vi "VerticalSpeedIndicator.vi"(6 "SignalSource":T2(ring), 7 "ScaleUnit(F=m/s; T=Ft/min/100)":bool, 8 "error in (no error)":errorcluster caption="Fehler (Eingang, kein Fehler)", 11 "SBG Data Cluster":T1) -> (0 "error out":errorcluster caption="Fehler (Ausgang)", 2 "VerticalSpeedDigital":dbl format="%.1f", 3 "VerticalSpeedIndicator":picture)   [LabVIEW 2023]
uses:
  SBG Data Cluster.ctl
  <vilib>/picture/picture.llb/imagedata.ctl
  <vilib>/Utility/miscctls.llb/LVBoundsTypeDef.ctl
panel:
  in  "Transparent":picture caption="Neue Grafik"
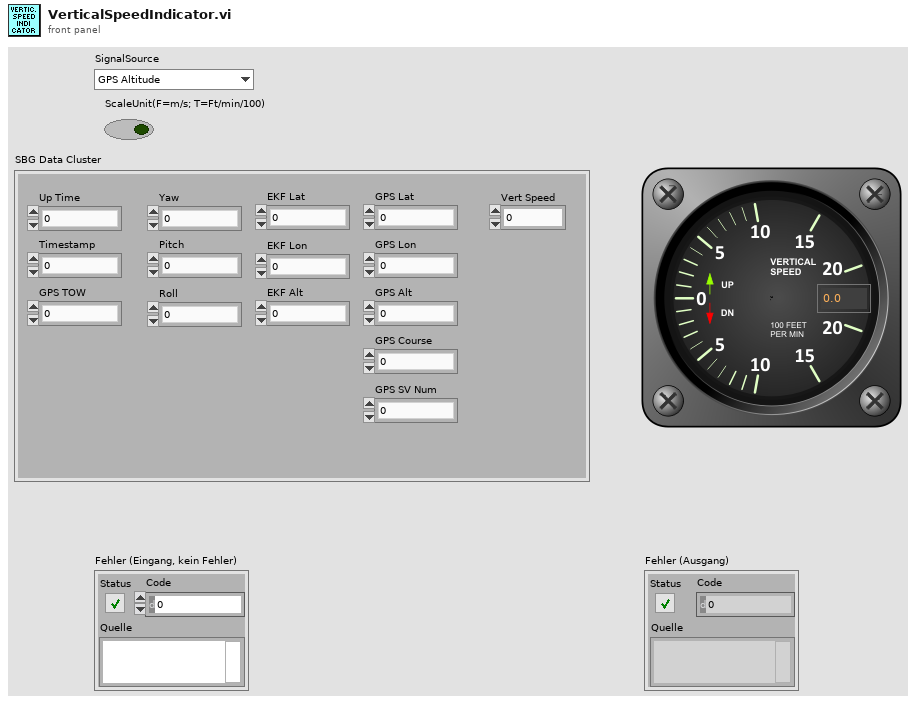
[diagram p1: front panel]
types:
  T1 = typedef "SBG Data Cluster.ctl" = cluster{"Up Time":u32, "Timestamp":u32, "Yaw":sgl, "Pitch":sgl, "Roll":sgl, "EKF Lat":dbl, "EKF Lon":dbl, "EKF Alt":dbl, "GPS Lat":dbl, "GPS Lon":dbl, "GPS Alt":dbl, "GPS Course":sgl, "GPS SV Num":u8, "GPS TOW":u32, "Vert Speed":dbl}
  T2 = enum16{"GPS Altitude", "Baro absolute Altitude", "Baro Vario"}
  T3 = typedef "LVBoundsTypeDef.ctl" = cluster{"Width":u32, "Height":u32}
  T4 = typedef "imagedata.ctl" = cluster{"image type":i32, "image depth":i32, "image":u8[], "mask":u8[], "colors":u32[], "Rectangle":cluster{"left":i16, "top":i16, "right":i16, "bottom":i16}}
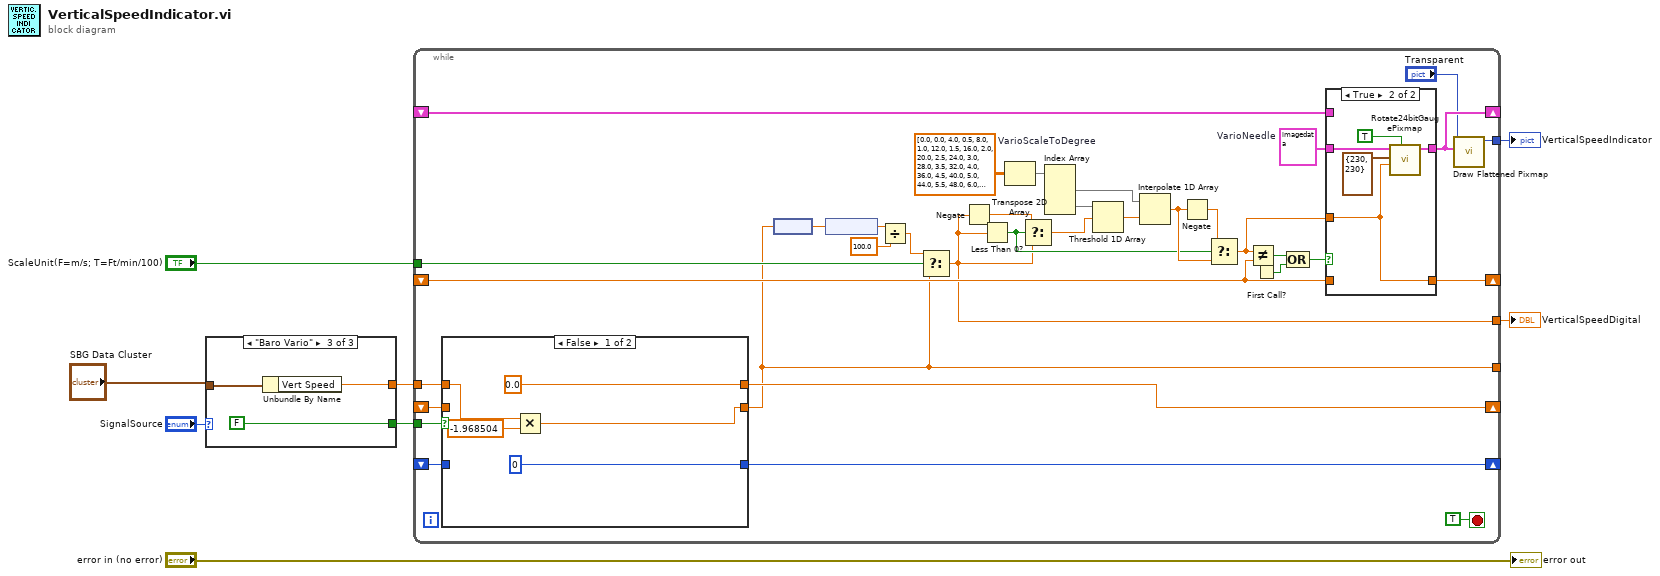
[diagram p0: block diagram]
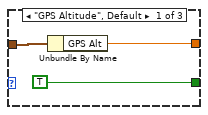
[diagram p2: hidden frame]
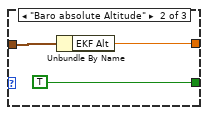
[diagram p3: hidden frame]
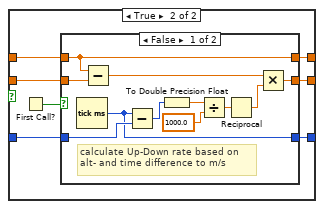
[diagram p4: hidden frame]
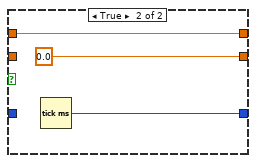
[diagram p5: hidden frame]
diagram:
  n1 = case shown="\"Baro Vario\"" "SignalSource" {
    tunnel: [TRUE TRUE FALSE] -> w3
    tunnel: "SBG Data Cluster" -> [w11 w14 w16]
    tunnel: [w10 w12 w15] -> w4
    frame "GPS Altitude", Default {
      n2 = Unbundle By Name(w11) -> ("GPS Alt"=w10:dbl)
    }
    frame "Baro absolute Altitude" {
      n3 = Unbundle By Name(w14) -> ("EKF Alt"=w12:dbl)
    }
    frame "Baro Vario" {
      n4 = Unbundle By Name(w16) -> ("Vert Speed"=w15:dbl)
    }
  }
  n5 = while {
    shift-right: [w50] -> _
    shift-left: _ -> [w44]
    shift-right: [w49] -> _
    shift-left: _ -> [w48]
    tunnel: [w46] -> w8
    tunnel: w4 -> [w23]
    tunnel: "ScaleUnit(F=m/s; T=Ft/min/100)" -> [w31]
    tunnel: [w18] -> w2
    tunnel: [w22] -> _
    shift-right: [w26] -> _
    shift-left: _ -> [w27]
    tunnel: w3 -> [w24]
    shift-right: [w21] -> _
    shift-left: _ -> [w20]
    stop <- TRUE stop-if-true
    w42 = dbl[][] [[0.0, 0.0], [4.0, 0.5], [8.0, 1.0], [12.0, 1.5], [16.0, 2.0], [20.0, 2.5], [24.0, 3.0], [28.0, 3.5], [32.0, 4.0], [36.0, 4.5], [40.0, 5.0], [44.0, 5.5], [48.0, 6.0], [52.0, 6.5], [56.0, 7.0], [60.0, 7.5], [64.0, 8.0], [68.0, 8.5], [72.0, 9.0], [76.0, 9.5], [80.0, 10.0], [88.0, 11.0], [96.0, 12.0], [104.0, 13.0], [112.0, 14.0], [120.0, 15.0], [128.0, 16.0], [136.0, 17.0], [144.0, 18.0], [152.0, 19.0], [160.0, 20.0]]  # VarioScaleToDegree
    w43 = T4 {"image type"=0, "image depth"=24, "image"=array[158700 elements], "mask"=[], "colors"=[], "Rectangle"={"left"=0, "top"=0, "right"=230, "bottom"=230}}  # VarioNeedle
    n6 = case shown="False" w24 {
      tunnel: w27 -> [_ w64]
      tunnel: [0.0 ("VerticalSpeed (m/s)") w63] -> w26
      tunnel: w23 -> [w55 w62]
      tunnel: [w53 w60] -> w22
      tunnel: [u32 0 ("millisecond timer value") w59] -> w21
      tunnel: w20 -> [_ w58]
      frame False {
        n7 = Multiply(x=w55, y=-1.968504) -> (x*y=w53:dbl)
      }
      frame True {
        n8 = First Call?() -> (First Call?: T/F=w61:bool)
        n9 = case shown="False" w61 {
          tunnel: w62 -> [w74 w78]
          tunnel: [w74 w78] -> w63
          tunnel: w64 -> [w75 _]
          tunnel: [w67 0.0] -> w60
          tunnel: [w72 w76] -> w59
          tunnel: w58 -> [w73 _]
          frame False {
            # "calculate Up-Down rate based on\nalt- and time difference to m/s"
            n10 = Tick Count (ms)() -> (millisecond timer value=w72:u32)
            n11 = Subtract(x=w74, y=w75) -> (x-y=w66:dbl)
            n12 = Subtract(x=w72, y=w73) -> (x-y=w71:u32)
            n13 = To Double Precision Float(number=w71) -> (double precision float=w70:dbl)
            n14 = Divide(x=w70, y=1000.0) -> (x/y=w68:dbl)
            n15 = Reciprocal(x=w68) -> (1/x=w65:dbl)
            n16 = Multiply(x=w66, y=w65) -> (x*y=w67:dbl)
          }
          frame True {
            n17 = Tick Count (ms)() -> (millisecond timer value=w76:u32)
          }
        }
      }
    }
    n18 = node(w22) -> (w30:dbl[unit])
    n19 = node(w30) -> (w29:dbl)
    n20 = Divide(x=w29, y=100.0) -> (x/y=w19:dbl)
    n21 = Select(t=w19, s=w31, f=w22) -> (s? t:f=w18:dbl)
    n22 = Negate(x=w18) -> (-x=w37:dbl)
    n23 = Less Than 0?(x=w18) -> (x < 0?=w39:bool)
    n24 = Transpose 2D Array(2D array=w42) -> (transposed array=w34:dbl[][])
    n25 = Select(t=w37, s=w39, f=w18) -> (s? t:f=w38:dbl)
    n26 = Index Array(array=w34) -> (element #1=w36:dbl[], element #2=w35:dbl[])  [unwired: 4 in]
    n27 = Threshold 1D Array(2:w38, 3:w35) -> (0:w33:dbl)  [unwired: 1 in]
    n28 = Interpolate 1D Array(1:w33, 2:w36) -> (0:w41:dbl)
    n29 = Negate(x=w41) -> (-x=w40:dbl)
    n30 = Select(t=w40, s=w39, f=w41) -> (s? t:f=w32:dbl)
    n31 = Not Equal?(x=w32, y=w44) -> (x != y?=w51:bool)
    n32 = First Call?() -> (First Call?: T/F=w25:bool)
    n33 = Compound Arithmetic op=OR(w51, w25) -> (w52:bool)
    n34 = case shown="True" w52 {
      tunnel: w43 -> [_ w85]
      tunnel: [w80 w84] -> w49
      tunnel: w48 -> [w80 _]
      tunnel: w44 -> [w79 _]
      tunnel: [w79 w82] -> w50
      tunnel: w32 -> [_ w82]
      frame False {
      }
      frame True {
        n35 = call "Rotate24bitGaugePixmap.vi"("Maske kombinieren? (F)"=TRUE, "Rotation Angle (degrees)"=w82, "Größe des Darstellungsbereichs"=T3 {"Width"=230, "Height"=230}, "image data"=w85) -> ("image data out"=w84:T4)  [unwired: 7 in]
      }
    }
    n36 = call <vilib>:"Draw Flattened Pixmap.vi"("image data"=w49, "picture"="Transparent") -> ("new picture"=w46:picture)  [unwired: 7 out]
  }
  "VerticalSpeedIndicator" <- w8
  "VerticalSpeedDigital" <- w2
  "error out" <- "error in (no error)"
